vi "Session Class.vi"() -> ()   [LabVIEW 2020]
uses:
  CTI/Session/Session.lvclass
panel:
  in  "CTI Session":refnum<class "Session.lvclass">
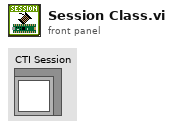
[diagram p1: front panel]
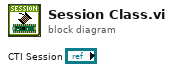
[diagram p0: block diagram]
diagram:
